vi "Draw_Picture from ImageData.vi"(11 "Image data in":T1) -> (2 "Icon":picture, 3 "Is default icon?":bool)   [LabVIEW 2021]
uses:
  <vilib>/picture/picture.llb/imagedata.ctl
  vi.lib/LabVIEW Icon API/lv_icon/lv_icon.lvlib
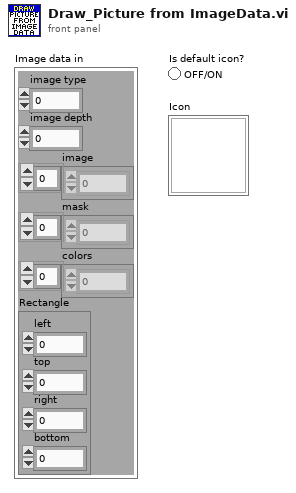
[diagram p1: front panel]
types:
  T1 = typedef "imagedata.ctl" = cluster{"image type":i32, "image depth":i32, "image":u8[], "mask":u8[], "colors":u32[], "Rectangle":cluster{"left":i16, "top":i16, "right":i16, "bottom":i16}}
  T2 = cluster{"left":i16, "top":i16, "right":i16, "bottom":i16}
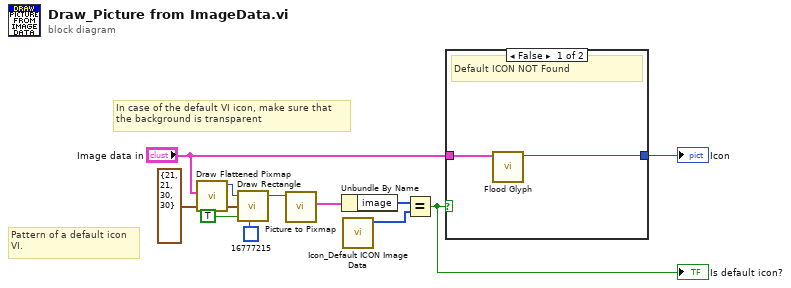
[diagram p0: block diagram]
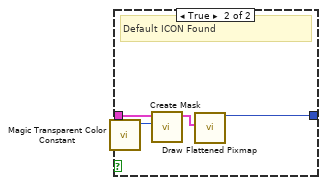
[diagram p2: hidden frame]
diagram:
  # "Pattern of a default icon\nVI."
  # "In case of the default VI icon, make sure that\nthe background is transparent"
  n1 = call <vilib>:"Draw Flattened Pixmap.vi"("image data"="Image data in") -> ("new picture"=w5:picture)  [unwired: 8 in]
  n2 = call <vilib>:"Draw Rectangle.vi"("picture"=w5, "rect"=T2 {"left"=21, "top"=21, "right"=30, "bottom"=30}, "fill?(F)"=TRUE, "color(black)"=u32 16777215) -> ("new picture"=w6:picture)  [unwired: 5 in]
  n3 = call <vilib>:"Picture to Pixmap.vi"("picture"=w6) -> ("image data"=w7:T1)  [unwired: 9 in, 1 out]
  n4 = Unbundle By Name(w7) -> ("image"=w9:u8[])
  n5 = call "Icon_Default ICON Image Data.vi"() -> ("DEFAULT ICON Image Data"=w10:u8[])  [unwired: 11 in]
  n6 = Equal?(x=w9, y=w10) -> (x = y?=w8:bool)
  "Is default icon?" <- w8
  n7 = case shown="False" w8 {
    tunnel: [w13 w16] -> w1
    tunnel: "Image data in" -> [w12 w17]
    frame False {
      # "Default ICON NOT Found"
      n8 = call "Flood Glyph.vi"("Image Data"=w12) -> ("Pic Out"=w13:picture)  [unwired: 1 in, 9 out]
    }
    frame True {
      # "Default ICON Found"
      n9 = call "Magic Transparent Color Constant.vi"() -> ("Magic transparent color constant"=w15:u32)  [unwired: 11 out]
      n10 = call <vilib>:"Create Mask.vi"("Mask Color (Black)"=w15, "image data"=w17) -> ("image data"=w14:T1)  [unwired: 9 in]
      n11 = call <vilib>:"Draw Flattened Pixmap.vi"("image data"=w14) -> ("new picture"=w16:picture)  [unwired: 8 in]
    }
  }
  "Icon" <- w1
